vi "CreateAc.vi"(0 "AnalogComparator":refnum<class "AnalogComparator.lvclass">, 5 "error in (no error)":errorcluster, 10 "AlarmType":T1=enum."Alarm", 12 "Tags":T2, 13 "Logger":refnum<class "Logger.lvclass">) -> (14 "AnalogComparator out":refnum<class "AnalogComparator.lvclass">, 19 "error out":errorcluster)   [LabVIEW 2019, in "AnalogComparator.lvclass"]
uses:
  AnalogComparator.lvclass
  D:/GIT H4000/H4000/src/Signal_class/Signal.lvclass
  Proccess_class/TAGs.ctl
  Logger_class/Logger.lvclass
  TypeDef/AlarmType.ctl
  AnalogComparator.lvclass/AnalogComparator.ctl
  Signal_class/Signal.lvclass
  Proccess_class/Proccess.lvclass
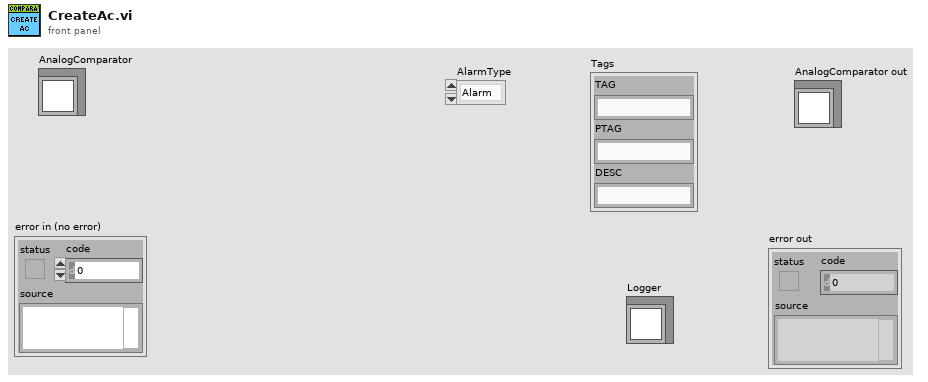
[diagram p1: front panel]
types:
  T1 = typedef "AlarmType.ctl" = enum16{"Normal", "Warning", "Alarm"}
  T2 = typedef "Proccess.lvclass/TAGs.ctl" = cluster{"TAG":string, "PTAG":string, "DESC":string}
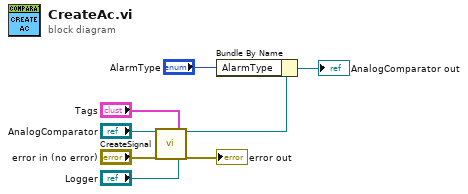
[diagram p0: block diagram]
diagram:
  n1 = call "CreateSignal.vi"("Signal in"="AnalogComparator", "error in (no error)"="error in (no error)", "Tags"="Tags", "Logger"="Logger") -> ("Signal out"=w3:refnum<class "AnalogComparator.lvclass">, "error out"=→"error out":errorcluster)  [unwired: 14 in]
  n2 = Bundle By Name(cluster=w3, "AlarmType"="AlarmType") -> (→"AnalogComparator out":refnum<class "AnalogComparator.lvclass">)
